vi "CC Convert DEC to String.vi"(8 "error in (no error)":errorcluster, 11 "DEC":dbl) -> (0 "error out":errorcluster, 2 "Declination":T1 {"Arc Sec" format="%0#2_6g"}, 3 "DEC String":string)   [LabVIEW 2021]
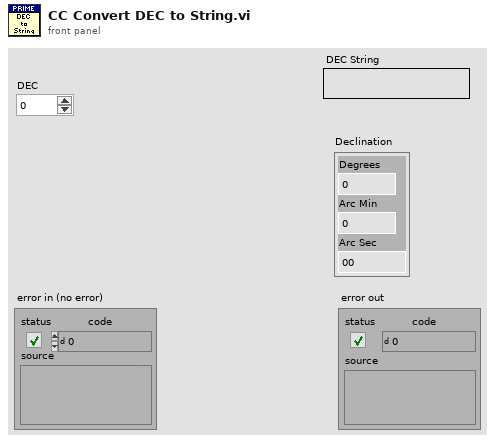
[diagram p1: front panel]
types:
  T1 = cluster{"Degrees":dbl, "Arc Min":dbl, "Arc Sec":dbl}
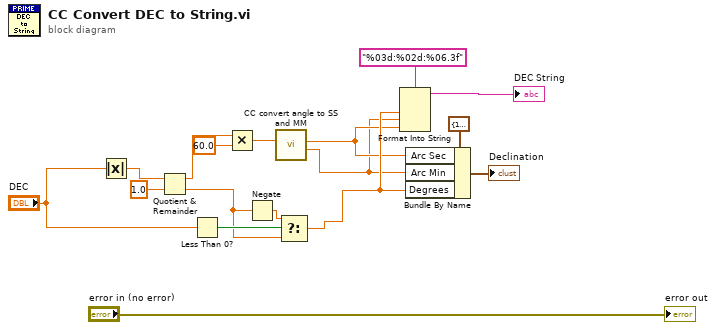
[diagram p0: block diagram]
diagram:
  n1 = Absolute Value(x="DEC") -> (abs(x)=w9:dbl)
  n2 = Quotient & Remainder(x=w9, y=1.0) -> (x-y*floor(x/y)=w15:dbl, floor(x/y)=w6:dbl)
  n3 = Less Than 0?(x="DEC") -> (x < 0?=w8:bool)
  n4 = Multiply(x=w15, y=60.0) -> (x*y=w3:dbl)
  n5 = Negate(x=w6) -> (-x=w7:dbl)
  n6 = call "CC convert angle to SS and MM.vi"("Angle"=w3) -> ("Minutes"=w1:dbl, "Seconds"=w2:dbl)  [unwired: 9 in]
  n7 = Select(t=w7, s=w8, f=w6) -> (s? t:f=w5:dbl)
  n8 = Format Into String(format string="%03d:%02d:%06.3f", w5, w1, w2) -> (resulting string=→"DEC String":string)  [unwired: 2 in, 1 out]
  n9 = Bundle By Name(cluster=T1 {"Degrees"=10.0, "Arc Min"=2.0, "Arc Sec"=11.040000000001555} ("Declination"), "Arc Sec"=w2, "Arc Min"=w1, "Degrees"=w5) -> (→"Declination":T1)
  "error out" <- "error in (no error)"
